vi "EstateMachine.vi"() -> ()   [LabVIEW 2020]
uses:
  <vilib>/ErrorRing/Error Ring.xnode
panel:
  out "Array 2":bool[](array[boolean])
  out "Array":dbl[](array[slide]) scale=0.0..100.0
  in  "Alarma":dbl(slide) scale=0.0..100.0
  in  "Formato":string(combo)
  out "String":string
  in  "Data_Analisis.Direccion":path
  in  "Stop":bool
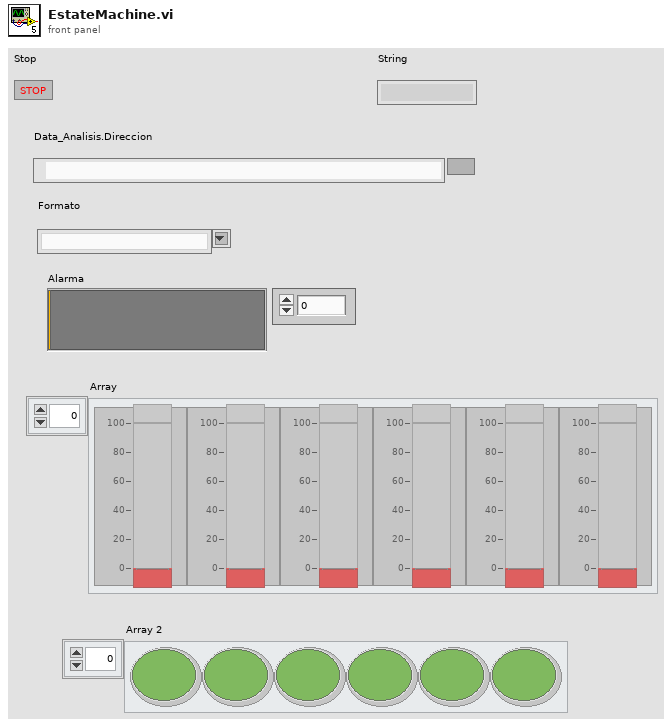
[diagram p1: front panel]
types:
  T1 = cluster{"Data_Analisis":cluster{"Direccion":path, "NombreArchivo":string, "Formato":string, "refnum out":refnum<file>}, "N values":cluster{"N_Elementos":i32, "L_min":dbl, "L_max":dbl}, "Hardware":cluster{"Data_Value":dbl[]}, "Warning":cluster{"Alarmas":bool[]}}
  T2 = cluster{"N_Elementos":i32, "L_min":dbl, "L_max":dbl}
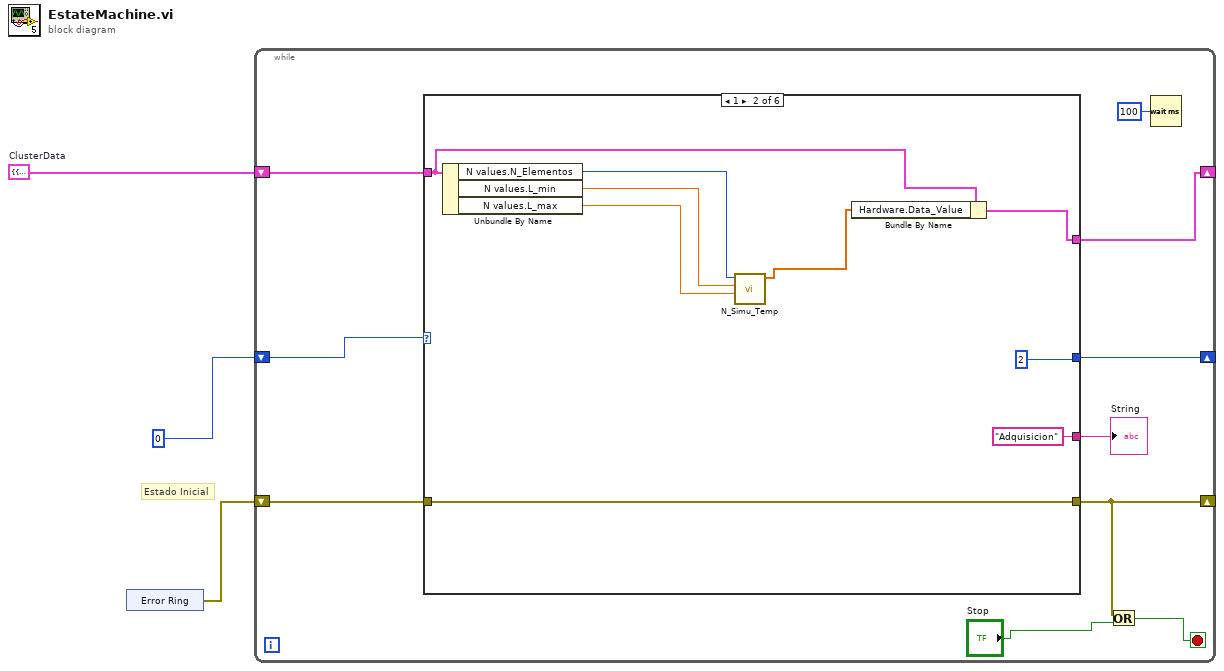
[diagram p0: block diagram]
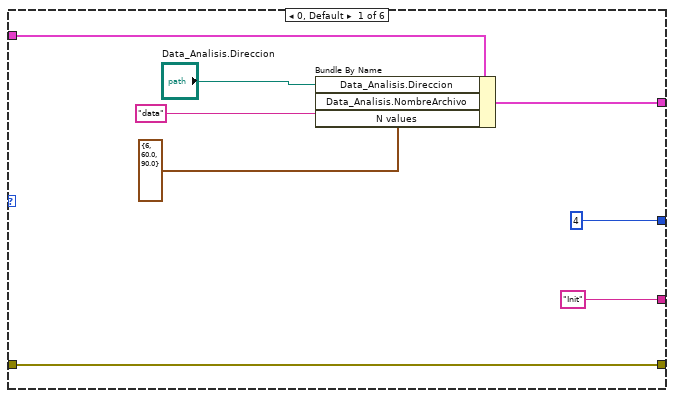
[diagram p2: hidden frame]
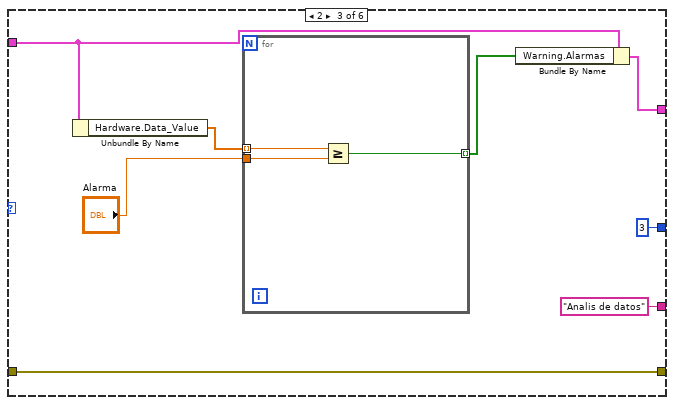
[diagram p3: hidden frame]
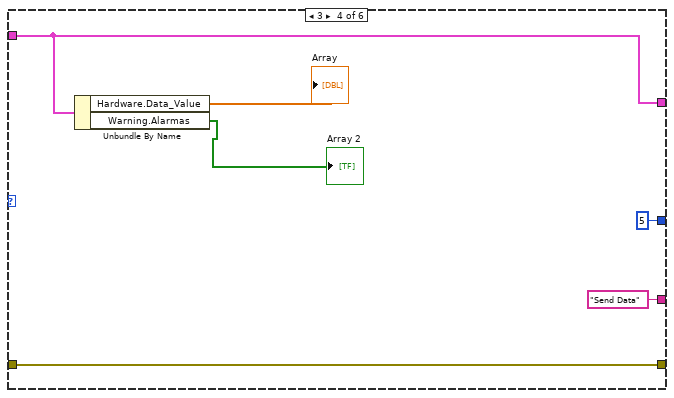
[diagram p4: hidden frame]
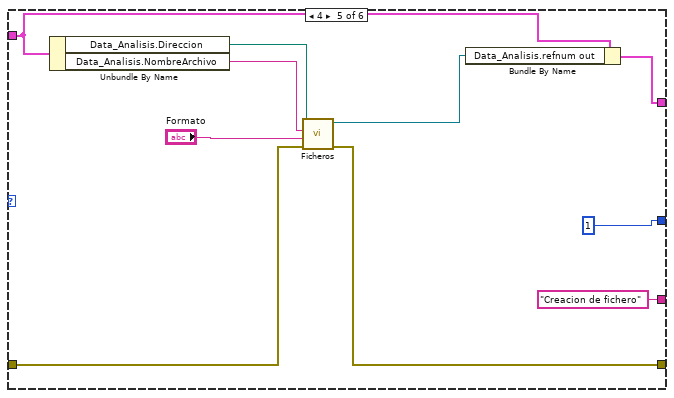
[diagram p5: hidden frame]
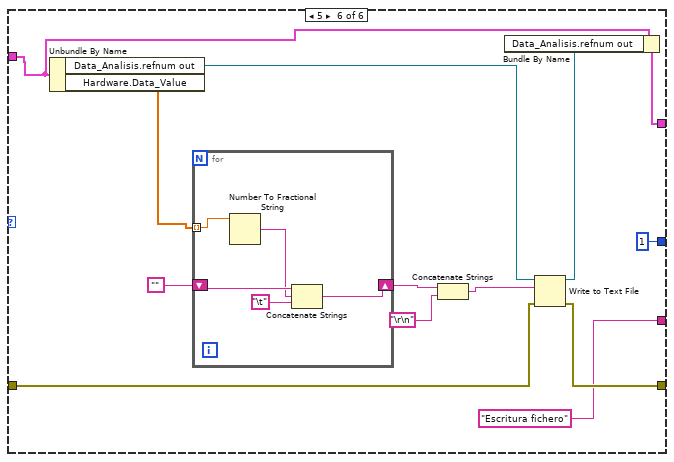
[diagram p6: hidden frame]
diagram:
  w3 = T1 {"Data_Analisis"={"Direccion"=path "", "NombreArchivo"="", "Formato"="", "refnum out"=refnum}, "N values"={"N_Elementos"=0, "L_min"=0.0, "L_max"=0.0}, "Hardware"={"Data_Value"=[]}, "Warning"={"Alarmas"=[]}}  # ClusterData
  # "Estado Inicial"
  n1 = xnode "Error Ring"() -> ("error out"=w1:errorcluster)
  n2 = while {
    shift-right: [w11] -> _
    shift-left: w3 -> [w12]
    shift-right: [w9] -> _
    shift-left: 0 -> [w13]
    shift-right: [w4] -> _
    shift-left: w1 -> [w10]
    stop <- w6 stop-if-true
    n3 = case shown="1" w13 {
      tunnel: w12 -> [w21 w26 w36 w45 w52 w61]
      tunnel: [w17 w24 w34 w45 w50 w62] -> w11
      tunnel: [w16 w27 w33 w44 w56 w63] -> w4
      tunnel: w10 -> [w16 w27 w33 w44 w57 w64]
      tunnel: [4 2 3 5 1 1] -> w9
      tunnel: ["Init" "Adquisicion" "Analis de datos" "Send Data" "Creacion de fichero" "Escritura fichero"] -> w8
      frame 0, Default {
        n4 = Bundle By Name(cluster=w21, "Data_Analisis.Direccion"="Data_Analisis.Direccion", "Data_Analisis.NombreArchivo"="data", "N values"=T2 {"N_Elementos"=6, "L_min"=60.0, "L_max"=90.0}) -> (w17:T1)
      }
      frame 1 {
        n5 = Unbundle By Name(w26) -> ("N values.N_Elementos"=w30:i32, "N values.L_min"=w29:dbl, "N values.L_max"=w28:dbl)
        n6 = call "N_Simu_Temp.vi"("Lmax"=w28, "Lmin"=w29, "Numeric"=w30) -> ("Array"=w25:dbl[])  [unwired: 8 in]
        n7 = Bundle By Name(cluster=w26, "Hardware.Data_Value"=w25) -> (w24:T1)
      }
      frame 2 {
        n8 = Unbundle By Name(w36) -> ("Hardware.Data_Value"=w38:dbl[])
        n9 = for {
          tunnel: w38 -> [w41] mode=indexing
          tunnel: "Alarma" -> [w40]
          tunnel: [w39] -> w35 mode=indexing
          n10 = Greater Or Equal?(x=w41, y=w40) -> (x >= y?=w39:bool)
        }
        n11 = Bundle By Name(cluster=w36, "Warning.Alarmas"=w35) -> (w34:T1)
      }
      frame 3 {
        n12 = Unbundle By Name(w45) -> ("Hardware.Data_Value"=→"Array":dbl[], "Warning.Alarmas"=→"Array 2":bool[])
      }
      frame 4 {
        n13 = Unbundle By Name(w52) -> ("Data_Analisis.Direccion"=w53:path, "Data_Analisis.NombreArchivo"=w54:string)
        n14 = call "Ficheros.vi"("error in (no error)"=w57, "Formato"="Formato", "Nombre Archivo"=w54, "Direccion"=w53) -> ("error out"=w56:errorcluster, "Byte Stream File out"=w51:refnum<file>)  [unwired: 6 in]
        n15 = Bundle By Name(cluster=w52, "Data_Analisis.refnum out"=w51) -> (w50:T1)
      }
      frame 5 {
        n16 = Unbundle By Name(w61) -> ("Data_Analisis.refnum out"=w65:refnum<file>, "Hardware.Data_Value"=w70:dbl[])
        n17 = for {
          tunnel: w70 -> [w75] mode=indexing
          shift-right: [w71] -> w68
          shift-left: "" -> [w74]
          n18 = Number To Fractional String(number=w75) -> (F-format string=w73:string)  [unwired: 3 in]
          n19 = Concatenate Strings(w74, w73, "\t") -> (w71:string)
        }
        n20 = Concatenate Strings(w68, "\r\n") -> (w66:string)
        n21 = Write to Text File(file (use dialog)=w65, text=w66, error in=w64) -> (refnum out=w60:refnum<file>, error out=w63:errorcluster)  [unwired: 1 in, 1 out]
        n22 = Bundle By Name(cluster=w61, "Data_Analisis.refnum out"=w60) -> (w62:T1)
      }
    }
    "String" <- w8
    n23 = Or(x=w4, y="Stop") -> (x .or. y?=w6:bool)
    n24 = Wait (ms)(milliseconds to wait=u32 100) -> ()  [unwired: 1 out]
  }
